vi "SignalAttrbGet.vi"(0 "MessageFrame":refnum<k21>="ESP_1\nLRA110") -> (14 "SignalsNameArry":string[](array[string]), 15 "ScaleFac":dbl[](array[numeric]), 16 "StartBitArry":u32[](array[numeric]), 17 "Length":u32[](array[numeric]), 18 "DataType":u32[](array[numeric]), 19 "DefaultValue":dbl[](array[numeric]))   [LabVIEW 2020]
uses:
  <resource>/objmgr/xnet.rc
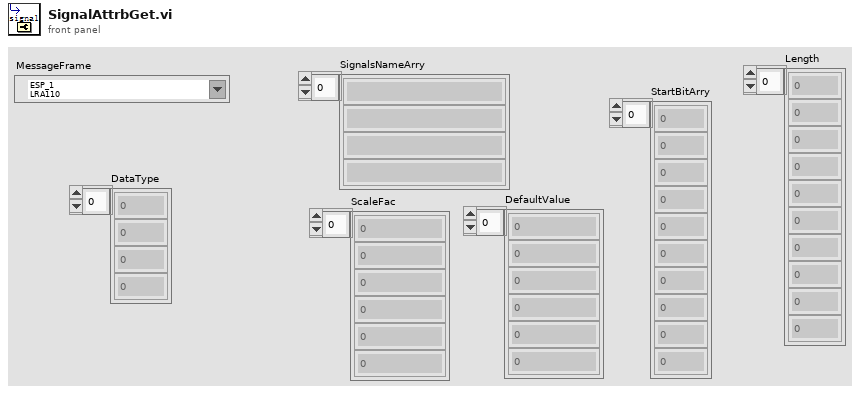
[diagram p1: front panel]
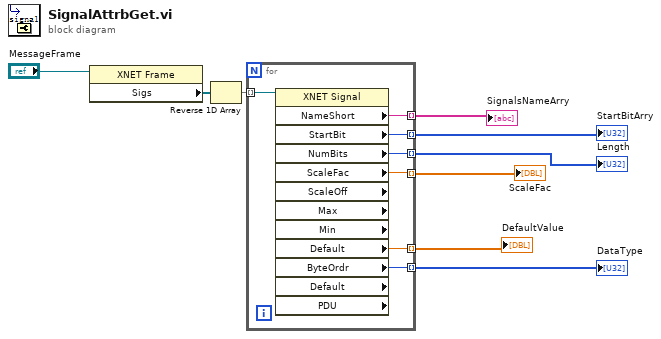
[diagram p0: block diagram]
diagram:
  n1 = property class="XNET Frame"(reference="MessageFrame") -> ("Sigs"=w8:refnum<k21>[])  [unwired: 1 in, 2 out]
  n2 = Reverse 1D Array(array=w8) -> (reversed array=w1:refnum<k21>[])
  n3 = for {
    tunnel: w1 -> [w16] mode=indexing
    tunnel: [w15] -> w6 mode=indexing
    tunnel: [w14] -> w7 mode=indexing
    tunnel: [w13] -> w5 mode=indexing
    tunnel: [w12] -> w3 mode=indexing
    tunnel: [w11] -> w4 mode=indexing
    tunnel: [w10] -> w2 mode=indexing
    n4 = property class="XNET Signal" props=["NameShort", "StartBit", "NumBits", "ScaleFac", "ScaleOff", "Max", "Min", "Default", "ByteOrdr", "Default", "PDU"](reference=w16) -> ("NameShort"=w15:string, "StartBit"=w12:u32, "NumBits"=w10:u32, "ScaleFac"=w14:dbl, "Default"=w13:dbl, "ByteOrdr"=w11:u32)  [unwired: 1 in, 7 out]
  }
  "SignalsNameArry" <- w6
  "ScaleFac" <- w7
  "DefaultValue" <- w5
  "StartBitArry" <- w3
  "DataType" <- w4
  "Length" <- w2
